vi "Get Cap.vi"(3 "error in":errorcluster, 4 "options":T1={"sp low"=0.0, "sp high"=100.0, "out low"=-100.0, "out high"=100.0, "hold (F)"=FALSE, "auto (T)"=TRUE, "pro. band (F)"=FALSE, "reverse acting (T)"=TRUE, "beta"=1.0, "linearity"=1.0, "dt (s)"=-1.0} {"dt (s)" format="%.2f"; "linearity" min=0.0 max=1.0 format="%.2f"; "sp low" format="%.2f"; "sp high" format="%.2f"; "out low" format="%.2f"; "out high" format="%.2f"; "beta" min=0.0 max=1.0 format="%.2f"}, 5 "VI Refnum 2":refnum<vi>) -> (1 "Setpoint (V)":dbl format="%.2f", 2 "VI Refnum":refnum<vi>)   [LabVIEW 2020]
panel:
  # "SP & PV range:"
  # "Output range:"
  # "-1: default,using\nsystem clock"
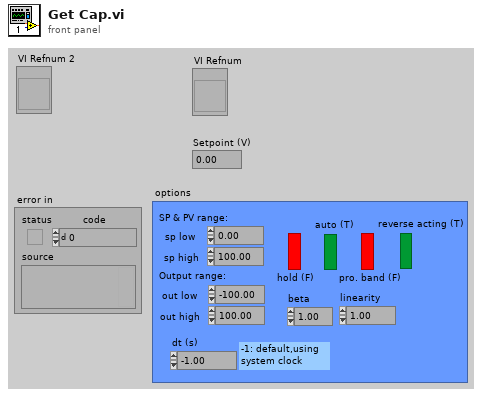
[diagram p1: front panel]
types:
  T1 = cluster{"sp low":dbl, "sp high":dbl, "out low":dbl, "out high":dbl, "hold (F)":bool, "auto (T)":bool, "pro. band (F)":bool, "reverse acting (T)":bool, "beta":dbl, "linearity":dbl, "dt (s)":dbl}
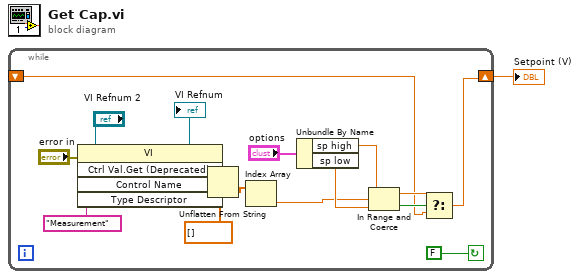
[diagram p0: block diagram]
diagram:
  n1 = while {
    shift-left: _ -> [w4]
    shift-right: [w3] -> w1
    stop <- FALSE continue-if-true
    n2 = invoke class="VI" method="Ctrl Val.Get (Deprecated)"(reference="VI Refnum 2", error in="error in", "Control Name"="Measurement") -> (reference out=→"VI Refnum":refnum<vi>, "Get Control Value"=w14:string)  [unwired: 2 in, 3 out]
    n3 = Unflatten From String(type=dbl[] [] ("Array Constant"), binary string=w14) -> (value=w13:dbl[])  [unwired: 3 in, 2 out]
    n4 = Index Array(array=w13) -> (element=w8:dbl)  [unwired: 1 in]
    n5 = Unbundle By Name("options") -> ("sp high"=w7:dbl, "sp low"=w9:dbl)
    n6 = In Range and Coerce(upper limit=w7, x=w8, lower limit=w9) -> (coerced(x)=w5:dbl, In Range?=w6:bool)
    n7 = Select(t=w5, s=w6, f=w4) -> (s? t:f=w3:dbl)
  }
  "Setpoint (V)" <- w1
